vi "Teleop.vi"(10 "Match Info":T1={"Autonomous Elapsed Seconds"=0.0, "TeleOp Elapsed Seconds"=0.0, "Disabled Elapsed Seconds"=0.0, "Visited Autonomous"=FALSE, "Visited TeleOp"=FALSE, "Visited Disabled"=FALSE, "Autonomous Settings"={"Autonomous Style"=enum."Independent", "VI Refnum"=refnum}}, 11 "Call Context":T2) -> ()   [LabVIEW 2012]
doc: "This VI is called for each TeleOp packet received from the DS where the robot is not disabled. It is often used to read from the joysticks and update I/O or to update setpoints for timed control loops. It should complete and return within 20 milliseconds or it may miss DS packets."
uses:
  <vilib>/Rock Robotics/WPI/DriverStation/WPI_DriverStationDerivedRobotMode.ctl
  <vilib>/Rock Robotics/WPI/DriverStation/WPI_DriverStationMatch Info.ctl
  <vilib>/Rock Robotics/WPI/DriverStation/DriverStationLCD/WPI_DriverStationLCDLCDLine.ctl
  Robot Global Data.vi
  <vilib>/Rock Robotics/WPI/RobotDrive/WPI_RobotDriveGetSetRefNum.vi
  <vilib>/Rock Robotics/WPI/Joystick/WPI_JoystickGetSetRefNum.vi
panel:
  in  "Buffer":string
  out "length":i32
  out "Numeric 1":dbl(slide) scale=0.0..100.0
  out "Boolean 2":bool
  out "Boolean 1":bool
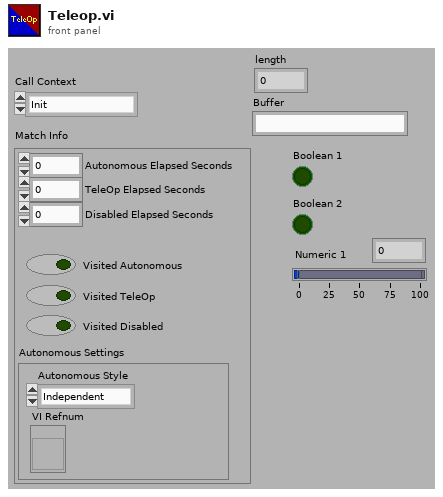
[diagram p1: front panel]
types:
  T1 = typedef "WPI_DriverStationMatch Info.ctl" = cluster{"Autonomous Elapsed Seconds":dbl, "TeleOp Elapsed Seconds":dbl, "Disabled Elapsed Seconds":dbl, "Visited Autonomous":bool, "Visited TeleOp":bool, "Visited Disabled":bool, "Autonomous Settings":cluster{"Autonomous Style":enum16{"Iterative", "Independent"}, "VI Refnum":refnum<vi>}}
  T2 = typedef "WPI_DriverStationDerivedRobotMode.ctl" = enum16{"Init", "Execute", "Stop"}
  T3 = typedef "WPI_DriverStationLCDLCDLine.ctl" = enum16{"Main - Line 1", "User - Line 2", "User - Line 3", "User - Line 4", "User - Line 5", "User - Line 6"}
  T4 = typedef "WPI_JoystickDevRef.ctl" = cluster{"Device":T5}
  T5 = typedef "WPI_JoystickDeviceEnum.ctl" = enum16{"USB 1", "USB 2", "USB 3", "USB 4", "Kinect 1", "Kinect 2"}
  T6 = typedef "WPI_SerialPortRef.ctl" = cluster{"DevStatus":errorcluster, "Serial Port Name":refnum<visa-resource-name>}
  T7 = typedef "WPI_RobotDriveDevRef.ctl" = cluster{"DevStatus":errorcluster, "Motors[]":T8[], "Square Inputs":bool, "Max Output":dbl, "Isochronous":bool}
  T8 = typedef "WPI_MotorControlDeviceRef.ctl" = cluster{"DeviceStatus":errorcluster, "Type":enum16{"PWM", "CAN"}, "PWM":cluster{"Digital Module":T9, "PWM Channel":T10, "DeadBand":T11}, "CAN":cluster{"Device Number":u8, "Control Mode":T12, "Semaphore":T13, "Max Vout":dbl}, "Invert":bool, "TransformRef":T14, "InvTransformRef":T14}
  T9 = typedef "FPGA_TypedefDigitalModule.ctl" = enum16{"Digital Module 1", "Digital Module 2"}
  T10 = typedef "FPGA_DIOPWMChannel.ctl" = enum8{"PWM 1", "PWM 2", "PWM 3", "PWM 4", "PWM 5", "PWM 6", "PWM 7", "PWM 8", "PWM 9", "PWM 10", "Invalid"}
  T11 = typedef "WPI_PWMDeadband.ctl" = cluster{"Name":string, "maxPositivePwm":i32, "minPositivePwm":i32, "centerPwm":i32, "maxNegativePwm":i32, "minNegativePwm":i32, "angularRange":u16}
  T12 = typedef "WPI_CANJaguar_ControlMode.ctl" = enum8{"Percent VBus", "Current", "Speed", "Position", "Voltage"}
  T13 = typedef "Semaphore RefNum" = refnum<k1>
  T14 = typedef "WPI_PWMTransform_ConPane.ctl" = refnum<vi>
  T15 = typedef "WPI_JoystickButtonState.ctl" = cluster{"Button 1":bool, "Button 2":bool, "Button 3":bool, "Button 4":bool, "Button 5":bool, "Button 6":bool, "Button 7":bool, "Button 8":bool, "Button 9":bool, "Button 10":bool, "Button 11":bool, "Button 12":bool}
  T16 = cluster{"axis 1 (x)":dbl, "axis 2 (y)":dbl, "axis 3 (throttle)":dbl, "axis 4":dbl, "axis 5":dbl, "axis 6":dbl}
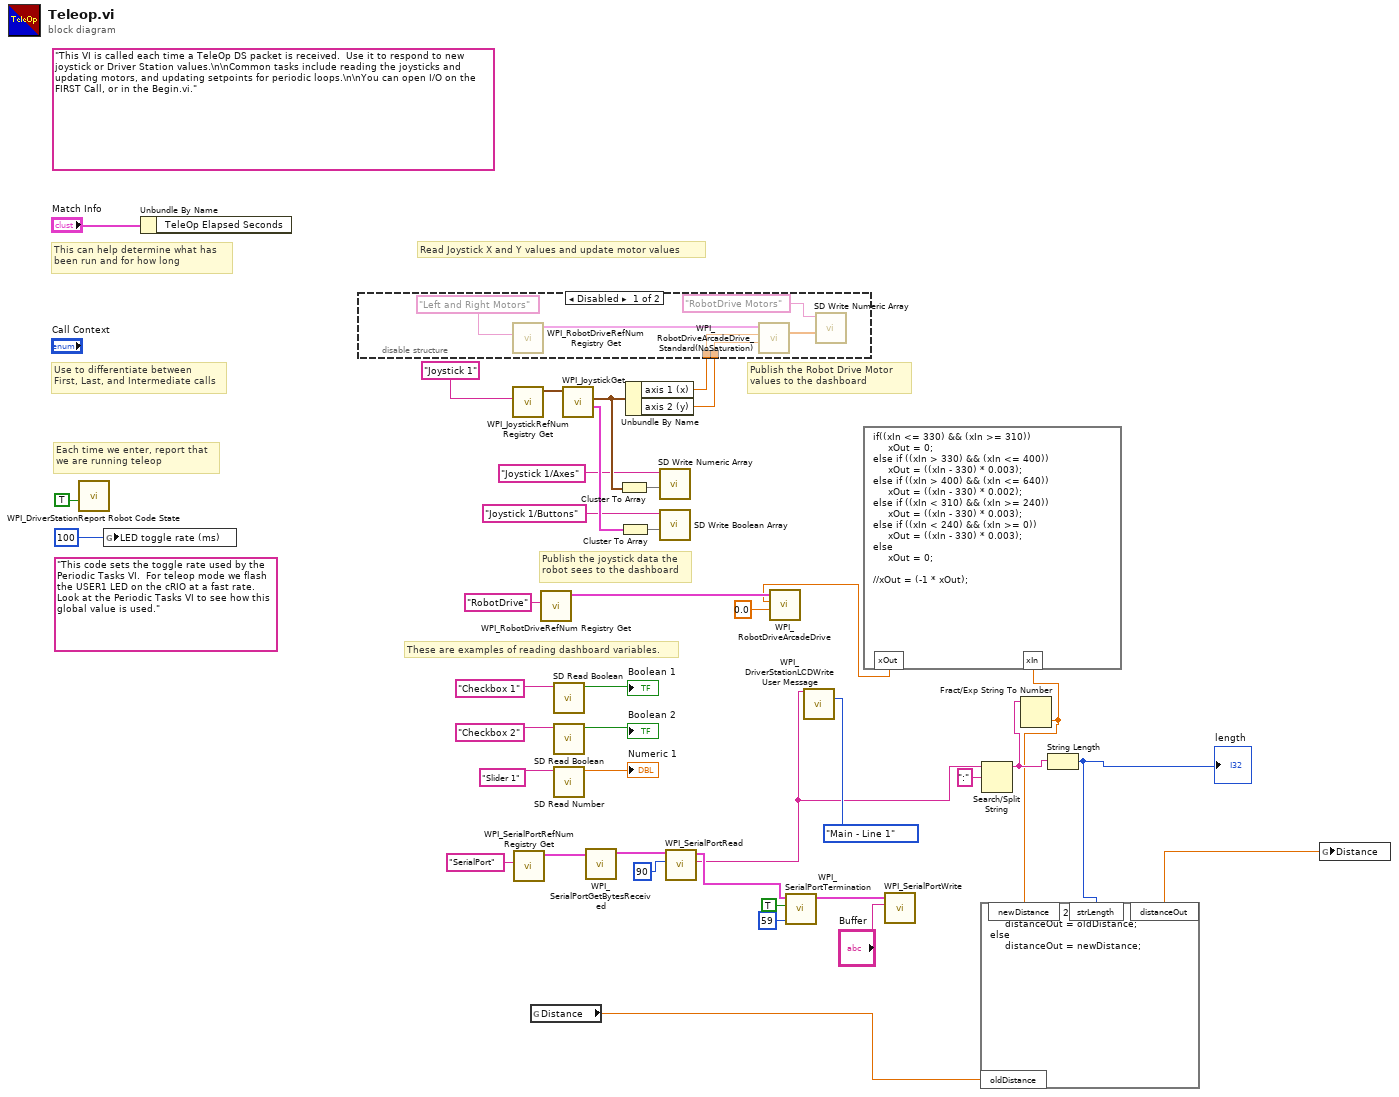
[diagram p0: block diagram]
diagram:
  (unwired) "This code sets the toggle rate used by the Periodic Tasks VI.  For teleop mode we flash the USER1 LED on the cRIO at a fast rate.  Look at the Periodic Tasks VI to see how this global value is used."
  (unwired) "This VI is called each time a TeleOp DS packet is received.  Use it to respond to new joystick or Driver Station values.\n\nCommon tasks include reading the joysticks and updating motors, and updating setpoints for periodic loops.\n\nYou can open I/O on the FIRST Call, or in the Begin.vi."
  # "Publish the Robot Drive Motor\nvalues to the dashboard"
  # "These are examples of reading dashboard variables."
  # "Publish the joystick data the\nrobot sees to the dashboard"
  # "Each time we enter, report that\nwe are running teleop"
  # "Use to differentiate between\nFirst, Last, and Intermediate calls"
  # "This can help determine what has\nbeen run and for how long"
  # "Read Joystick X and Y values and update motor values"
  n1 = call <vilib>:"WPI_DriverStationReport Robot Code State.vi"("TeleOp"=TRUE ("Autonomous")) -> ()  [unwired: 10 in, 1 out]
  n2 = global write "Robot Global Data.vi" "LED toggle rate (ms)"(u32 100 ("LED ms toggle rate")) -> ()
  n3 = Unbundle By Name("Match Info") -> ()  [unwired: 1 out]
  n4 = call <vilib>:"WPI_JoystickRefNum Registry Get.vi"("refnum name"="Joystick 1") -> ("JoystickDevRef"=w38:T4)  [unwired: 1 in, 9 out]
  n5 = call <vilib>:"WPI_SerialPortRefNum Registry Get.vi"("refnum name"="SerialPort") -> ("SerialPortRef"=w18:T6)  [unwired: 9 in, 1 out]
  n6 = global read "Robot Global Data.vi" "Distance"() -> (w3:dbl)
  n7 = call <vilib>:"WPI_RobotDriveRefNum Registry Get.vi"("refnum name"="RobotDrive") -> ("RobotDriveDevRef"=w22:T7)  [unwired: 9 in, 1 out]
  n8 = call <vilib>:"SD Read Boolean.vi"("Name"="Checkbox 1" ("refnum name")) -> ("Boolean"=→"Boolean 1":bool)  [unwired: 8 in, 2 out]
  n9 = call <vilib>:"SD Read Boolean.vi"("Name"="Checkbox 2" ("refnum name")) -> ("Boolean"=→"Boolean 2":bool)  [unwired: 8 in, 2 out]
  n10 = call <vilib>:"SD Read Number.vi"("Name"="Slider 1" ("refnum name")) -> ("Numeric"=→"Numeric 1":dbl)  [unwired: 8 in, 2 out]
  n11 = call <vilib>:"WPI_JoystickGet.vi"("JoystickDevRef"=w38) -> ("Buttons"=w35:T15, "Axes"=w32:T16)  [unwired: 1 in, 4 out]
  n12 = call <vilib>:"WPI_SerialPortGetBytesReceived.vi"("SerialPortRef"=w18) -> ("SerialPortRef"=w17:T6)  [unwired: 8 in, 2 out]
  n13 = Cluster To Array(cluster=w32) -> (array=w31:dbl[])
  n14 = Cluster To Array(cluster=w35) -> (array=w34:bool[])
  n15 = Unbundle By Name(w32) -> ("axis 1 (x)"=w21:dbl, "axis 2 (y)"=w20:dbl)
  n16 = disable-structure shown="Disabled" {
    disable-tunnel: w21 -> [w44 _]
    disable-tunnel: w20 -> [w43 _]
    frame Disabled {
      n17 = call <vilib>:"WPI_RobotDriveRefNum Registry Get.vi"("refnum name"="Left and Right Motors") -> ("RobotDriveDevRef"=w45:T7)  [unwired: 1 in, 9 out]
      n18 = call <vilib>:"WPI_RobotDriveArcadeDrive_Standard(NoSaturation).vi"("Y axis value"=w43, "X axis value"=w44, "RobotDriveDevRef"=w45) -> ("Motor Values"=w41:dbl[])  [unwired: 1 in, 7 out]
      n19 = call <vilib>:"SD Write Numeric Array.vi"("Numeric Array"=w41, "Name"="RobotDrive Motors") -> ()  [unwired: 8 in, 2 out]
    }
    frame Enabled {
    }
  }
  n20 = call <vilib>:"SD Write Numeric Array.vi"("Numeric Array"=w31, "Name"="Joystick 1/Axes") -> ()  [unwired: 8 in, 2 out]
  n21 = call <vilib>:"SD Write Boolean Array.vi"("Boolean Array"=w34, "Name"="Joystick 1/Buttons") -> ()  [unwired: 8 in, 2 out]
  n22 = call <vilib>:"WPI_SerialPortRead.vi"("Num Bytes to Read"=u32 90, "SerialPortRef"=w17) -> ("Buffer"=w10:string, "SerialPortRef"=w15:T6)  [unwired: 7 in, 1 out]
  n23 = call <vilib>:"WPI_SerialPortTermination.vi"("Termination Char (0xA = '\\n' = LF)"=u8 59 ("Termination Char (0xA = '\\n' = LF)"), "Enable? (T)"=TRUE, "SerialPortRef"=w15) -> ("SerialPortRef"=w6:T6)  [unwired: 7 in, 1 out]
  n24 = call <vilib>:"WPI_DriverStationLCDWrite User Message.vi"("line text"=w10, "line"=WPI_DriverStationLCDLCDLine."Main - Line 1") -> ()  [unwired: 13 in, 1 out]
  n25 = call <vilib>:"WPI_SerialPortWrite.vi"("Buffer"="Buffer", "SerialPortRef"=w6) -> ()  [unwired: 7 in, 3 out]
  n26 = Search/Split String(string=w10, search string/char (-)=":") -> (substring before match=w7:string)  [unwired: 1 in, 2 out]
  n27 = Fract/Exp String To Number(string=w7) -> (number=w1:dbl)  [unwired: 3 in, 1 out]
  n28 = formula code="if((xIn <= 330) && (xIn >= 310))\n     xOut = 0;\nelse if ((xIn > 330) && (xIn <= 400))\n     xOut = ((xIn - 330) * 0.003);\nelse if ((xIn > 400) && (xIn <= 640))\n     xOut = ((xIn - 330) * 0.002);\nelse if ((xIn < 310) && (xIn >= 240))\n     xOut = ((xIn - 330) * 0.003);\nelse if ((xIn < 240) && (xIn >= 0))\n     xOut = ((xIn - 330) * 0.003);\nelse\n     xOut = 0;\n\n//xOut = (-1 * xOut);"("xIn"=w1) -> ("xOut"=w8:dbl)
  n29 = call-poly <vilib>:"WPI_RobotDriveArcadeDrive.vi"("Y axis value"=0.0, "X axis value"=w8, "RobotDriveDevRef"=w22) -> ()  [unwired: 6 in, 3 out]
  n30 = String Length(string=w7) -> (length=w4:i32)
  "length" <- w4
  n31 = formula code="if (strLength < 2) \n     distanceOut = oldDistance;\nelse\n     distanceOut = newDistance;"("strLength"=w4, "oldDistance"=w3, "newDistance"=w1) -> ("distanceOut"=w2:dbl)
  n32 = global write "Robot Global Data.vi" "Distance"(w2) -> ()
